vi "char match position v0.3.vi"(1 "StringIn":string="0407P311.0.00T", 2 "matching character(s)":string) -> (0 "last matching position":i32)   [LabVIEW 2020]
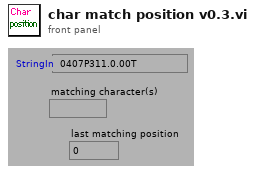
[diagram p1: front panel]
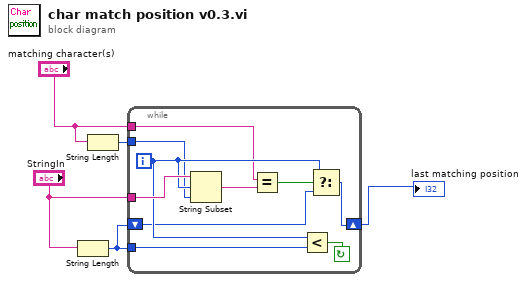
[diagram p0: block diagram]
diagram:
  n1 = String Length(string="StringIn") -> (length=w1:i32)
  n2 = String Length(string="matching character(s)") -> (length=w2:i32)
  n3 = while {
    tunnel: w2 -> [w6]
    tunnel: "matching character(s)" -> [w7]
    shift-left: w1 -> [w9]
    shift-right: [w10] -> w4
    tunnel: "StringIn" -> [w13]
    tunnel: w1 -> [w14]
    i -> [w11]
    stop <- w15 continue-if-true
    n4 = String Subset(string=w13, offset (0)=w11, length (rest)=w6) -> (substring=w8:string)
    n5 = Equal?(x=w7, y=w8) -> (x = y?=w12:bool)
    n6 = Less?(x=w11, y=w14) -> (x < y?=w15:bool)
    n7 = Select(t=w11, s=w12, f=w9) -> (s? t:f=w10:i32)
  }
  "last matching position" <- w4
